vi "IRH3T.vi"(8 "Due Dates":u16[](array[numeric]), 9 "Initial Tardiness":i32, 10 "Schedule 2B Improved":u16[](array[numeric]), 11 "Proocessing Times  (Machines x Jobs)":u16[][](array[numeric])=[[208, 80, 8, 184, 218, 197, 100, 5], [64, 30, 39, 91, 257, 38, 34, 447], [23, 215, 125, 135, 165, 136, 164, 37], [88, 22, 207, 5, 58, 213, 52, 355], [6, 181, 111, 222, 27, 259, 91, 103], [149, 37, 22, 14, 71, 155, 536, 16], [113, 71, 274, 348, 187, 1, 3, 3], [349, 364, 214, 1, 17, 1, 20, 34]]) -> (1 "IRH3T Schedule Out":u16[](array[numeric]), 2 "Total Tardiness":u16, 3 "IRH3T (Reordered) Schedule Out":u16[](array[numeric]))   [LabVIEW 2013]
uses:
  Classes/Scheduler_Class/Operation to Machine Job Tuple.vi
  Classes/Scheduler.lvclass
panel:
  out "Equal?":bool
  out "Job Completion Times":u16[](array[numeric])
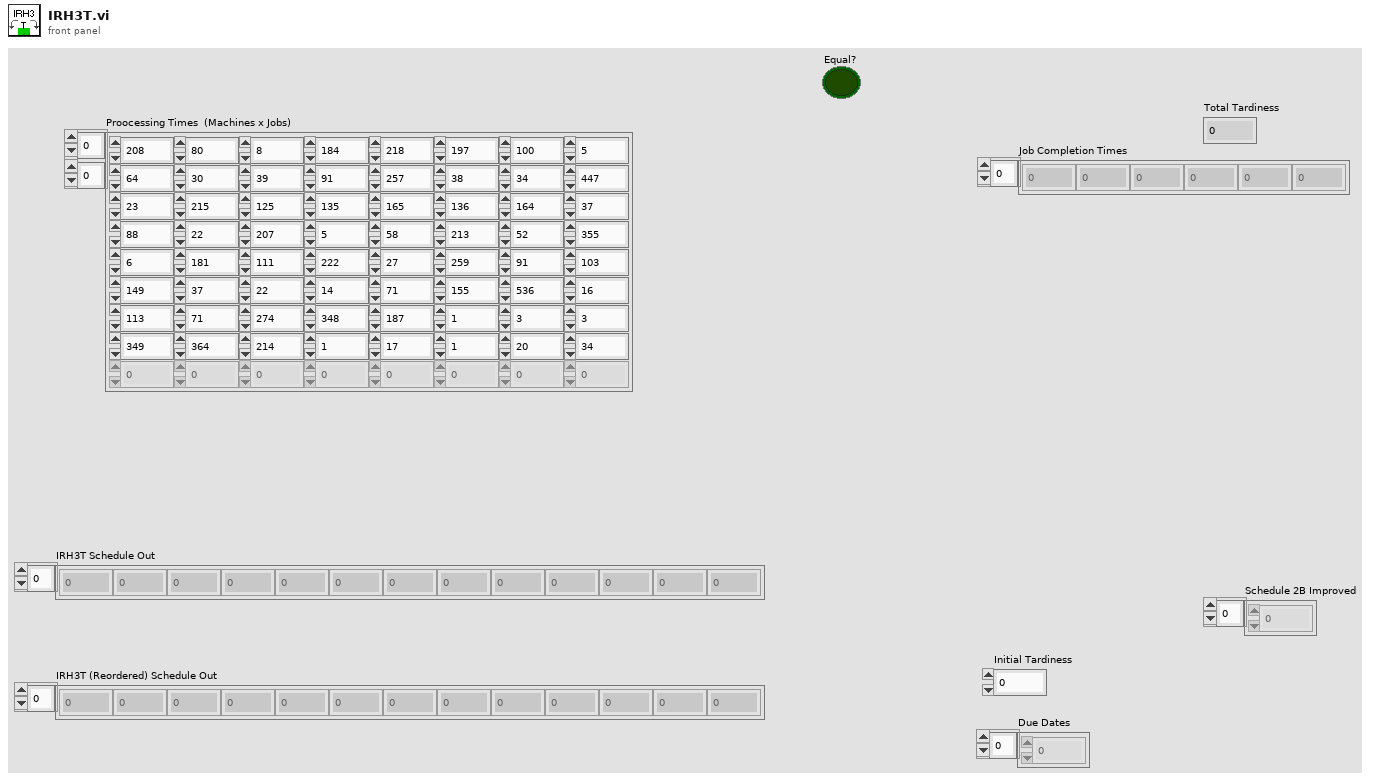
[diagram p1: front panel]
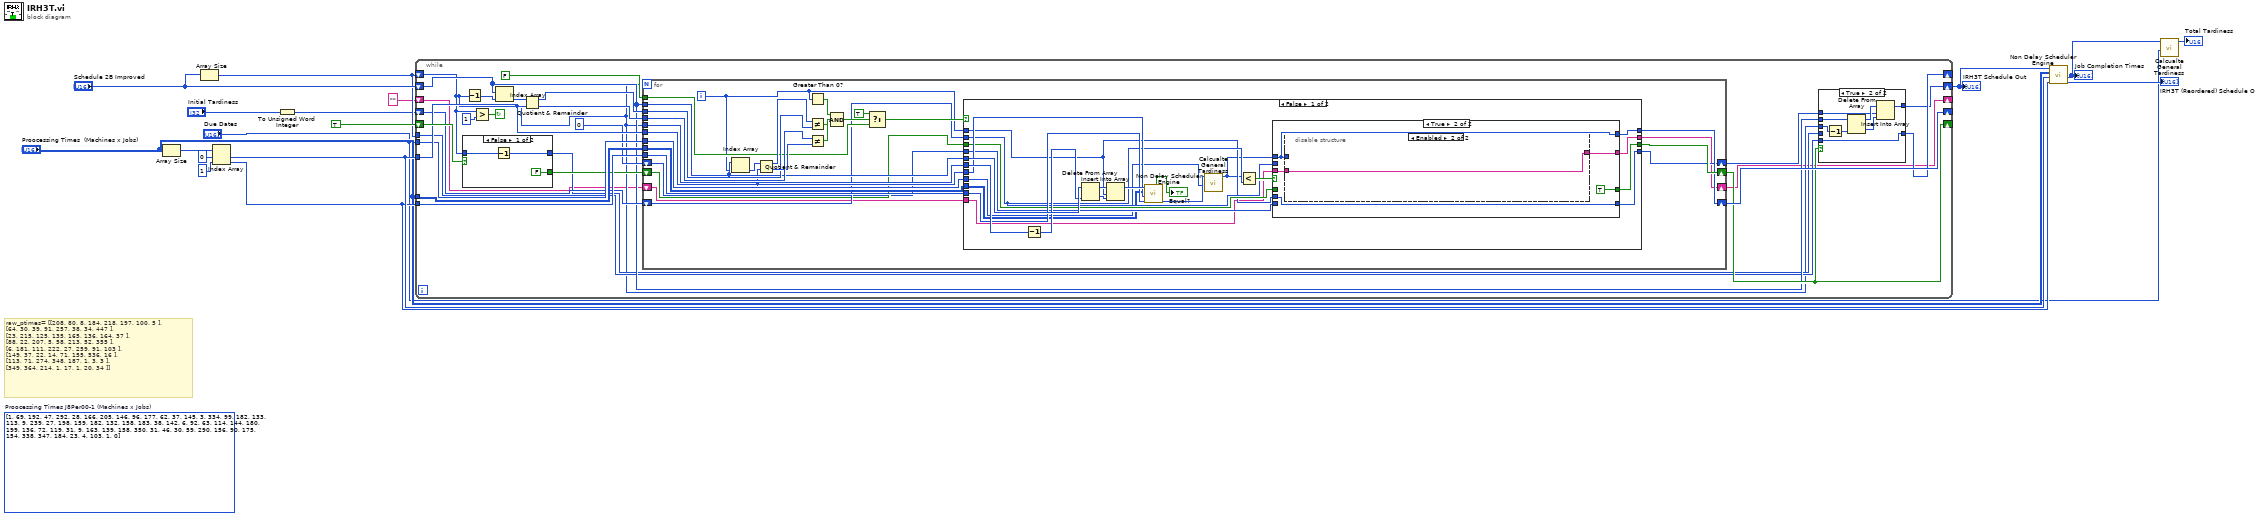
[diagram p0: block diagram]
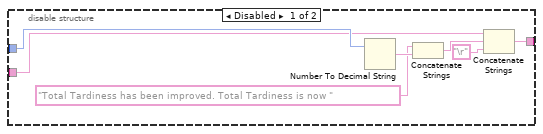
[diagram p4: hidden frame]
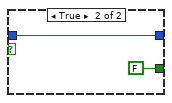
[diagram p6: hidden frame]
diagram:
  (unwired) u16[][] [[1, 69, 192, 47, 292, 28, 166, 205], [146, 96, 177, 62, 37, 145, 3, 334], [99, 182, 133, 113, 9, 239, 27, 198], [159, 182, 132, 158, 183, 38, 142, 6], [92, 63, 114, 144, 180, 199, 136, 72], [119, 31, 9, 163, 139, 158, 350, 31], [46, 30, 59, 290, 156, 90, 175, 154], [338, 347, 184, 23, 4, 103, 1, 0]]  # Proocessing Times J8Per00-1 (Machines x Jobs)
  # "raw_ptimes= [[208, 80, 8, 184, 218, 197, 100, 5 ],\n[64, 30, 39, 91, 257, 38, 34, 447 ],\n[23, 215, 125, 135, 165, 136, 164, 37 ],\n[88, 22, 207, 5, 58, 213, 52, 355 ],\n[6, 181, 111, 222, 27, 259, 91, 103 ],\n[149, 37, 22, 14, 71, 155, 536, 16 ],\n[113, 71, 274, 348, 187, 1, 3, 3 ],\n[349, 364, 214, 1, 17, 1, 20, 34 ]]"
  n1 = Array Size(array="Proocessing Times  (Machines x Jobs)") -> (size(s)=w15:i32[])
  n2 = Array Size(array="Schedule 2B Improved") -> (size(s)=w12:i32)
  n3 = Index Array(array=w15, index #1=0 ("index"), index #2=1 ("index")) -> (element #1=w10:i32, element #2=w9:i32)
  n4 = To Unsigned Word Integer(number="Initial Tardiness") -> (unsigned 16bit integer=w1:u16)
  n5 = while {
    shift-right: [w23] -> _
    shift-left: w12 -> [w21]
    shift-right: [w27] -> _
    shift-left: TRUE -> [w41]
    tunnel: w10 -> [w37]
    tunnel: "Proocessing Times  (Machines x Jobs)" -> [w34]
    tunnel: w9 -> [w33]
    tunnel: "Due Dates" -> [w32]
    shift-right: [w29] -> _
    shift-left: w1 -> [w31]
    shift-right: [w20] -> w11
    shift-left: "Schedule 2B Improved" -> [w26]
    tunnel: w12 -> [w24]
    shift-right: [w18] -> _
    shift-left: "" -> [w19]
    stop <- w42 continue-if-true
    n6 = case shown="False" w41 {
      tunnel: w21 -> [w127 w129]
      tunnel: [w126 w129] -> w22
      tunnel: [FALSE FALSE] -> w30
      frame False {
        n7 = Decrement(x=w127) -> (x-1=w126:i32)
      }
      frame True {
      }
    }
    n8 = Decrement(x=w21) -> (x-1=w40:i32)
    n9 = Greater?(x=w21, y=1) -> (0:w42:bool)
    n10 = Index Array(array=w26, index=w40) -> (element=w39:u16)
    n11 = Quotient & Remainder(x=w39, y=w37) -> (x-y*floor(x/y)=w36:i32, floor(x/y)=w35:i32)
    n12 = for {
      N: w21 -> [_]
      tunnel: FALSE -> [w71]
      tunnel: w26 -> [w68]
      tunnel: w37 -> [w64]
      tunnel: w36 -> [w74]
      tunnel: w35 -> [w78]
      tunnel: w21 -> [w67]
      tunnel: w34 -> [w65]
      tunnel: w33 -> [w63]
      tunnel: w32 -> [w62]
      shift-right: [w59] -> w27
      shift-left: w30 -> [w60]
      shift-right: [w58] -> w29
      shift-left: w31 -> [w61]
      shift-right: [w56] -> w25
      shift-left: 0 -> [w57]
      shift-right: [w54] -> w18
      shift-left: w19 -> [w55]
      i -> [w66]
      n13 = Index Array(array=w68, index=w66) -> (element=w80:u16)
      n14 = Quotient & Remainder(x=w80, y=w64) -> (x-y*floor(x/y)=w75:i32, floor(x/y)=w77:i32)
      n15 = Greater Than 0?(x=w66) -> (x > 0?=w79:bool)
      n16 = Not Equal?(x=w75, y=w74) -> (x != y?=w73:bool)
      n17 = Not Equal?(x=w78, y=w77) -> (x != y?=w76:bool)
      n18 = Compound Arithmetic op=AND(w79, w76, w73) -> (w72:bool)
      n19 = Select(t=TRUE, s=w72, f=w71) -> (s? t:f=w69:bool)
      n20 = case shown="False" w69 {
        tunnel: w68 -> [w103 _]
        tunnel: w67 -> [w102 _]
        tunnel: w66 -> [w89 _]
        tunnel: w65 -> [w86 _]
        tunnel: w64 -> [w98 _]
        tunnel: w63 -> [w97 _]
        tunnel: w62 -> [w83 _]
        tunnel: w61 -> [w92 w123]
        tunnel: w60 -> [w95 w124]
        tunnel: [w94 w124] -> w59
        tunnel: [w93 w123] -> w58
        tunnel: w57 -> [w91 w122]
        tunnel: [w90 w122] -> w56
        tunnel: w55 -> [w88 w121]
        tunnel: [w87 w121] -> w54
        frame False {
          n21 = Decrement(x=w102) -> (x-1=w101:i32)
          n22 = Delete From Array(array=w103, index=w101) -> (deleted portion=w85:u16, array with subset deleted=w100:u16[])  [unwired: 1 in]
          n23 = Insert Into Array(array=w100, index=w89, new element=w85) -> (w99:u16[])
          n24 = call "Non Delay Scheduler Engine.vi"("Number of  Jobs"=w97, "Number of Machines"=w98, "Processing Times"=w86, "Schedule"=w99) -> ("Reordered Schedule"=w84:u16[], "Equal?"=→"Equal?":bool)  [unwired: 2 in, 4 out]
          n25 = call "Calcualte General Tardiness.vi"("Due Dates"=w83, "Job Completion Times"=w84) -> ("Total Tardiness (U16)"=w82:u16)  [unwired: 9 in]
          n26 = Less?(x=w82, y=w92) -> (x < y?=w96:bool)
          n27 = case shown="True" w96 {
            tunnel: [w107 TRUE] -> w94
            tunnel: w95 -> [w107 _]
            tunnel: w82 -> [_ w110]
            tunnel: [w106 w110] -> w93
            tunnel: w92 -> [w106 _]
            tunnel: w91 -> [w105 _]
            tunnel: [w105 w111] -> w90
            tunnel: w89 -> [_ w111]
            tunnel: w88 -> [w104 w109]
            tunnel: [w104 w108] -> w87
            frame False {
            }
            frame True {
              n28 = disable-structure shown="Enabled" {
                disable-tunnel: w110 -> [w119 _]
                disable-tunnel: w109 -> [w116 w120]
                disable-tunnel: [w113 w120] -> w108
                frame Disabled {
                  n29 = Number To Decimal String(number=w119) -> (decimal integer string=w118:string)  [unwired: 1 in]
                  n30 = Concatenate Strings("Total Tardiness has been improved. Total Tardiness is now ", w118) -> (w115:string)
                  n31 = Concatenate Strings(w116, w115, "\r") -> (w113:string)
                }
                frame Enabled {
                }
              }
            }
          }
        }
        frame True {
        }
      }
    }
    n32 = case shown="True" w27 {
      tunnel: w26 -> [w44 w53]
      tunnel: w21 -> [_ w51]
      tunnel: w25 -> [_ w49]
      tunnel: [w45 w47] -> w23
      tunnel: w24 -> [_ w47]
      tunnel: w22 -> [w45 _]
      tunnel: [w44 w46] -> w20
      frame False {
      }
      frame True {
        n33 = Decrement(x=w51) -> (x-1=w52:i32)
        n34 = Delete From Array(array=w53, index=w52) -> (deleted portion=w48:u16, array with subset deleted=w50:u16[])  [unwired: 1 in]
        n35 = Insert Into Array(array=w50, index=w49, new element=w48) -> (w46:u16[])
      }
    }
  }
  "IRH3T Schedule Out" <- w11
  n36 = call "Non Delay Scheduler Engine.vi"("Number of  Jobs"=w9, "Number of Machines"=w10, "Processing Times"="Proocessing Times  (Machines x Jobs)", "Schedule"=w11) -> ("Reordered Schedule"=→"IRH3T (Reordered) Schedule Out":u16[], "Job Completion Times"=w5:u16[])  [unwired: 2 in, 4 out]
  "Job Completion Times" <- w5
  n37 = call "Calcualte General Tardiness.vi"("Due Dates"="Due Dates", "Job Completion Times"=w5) -> ("Total Tardiness (U16)"=→"Total Tardiness":u16)  [unwired: 9 in]
